vi "RT Variable Test.vi"() -> ()   [LabVIEW 2015]
panel:
  out "Log?":bool
  out "Operating?":bool
  out "a":dbl
  in  "stop":bool
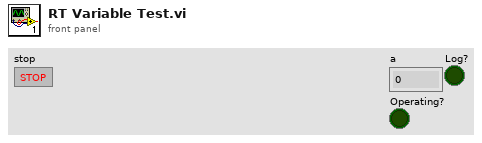
[diagram p1: front panel]
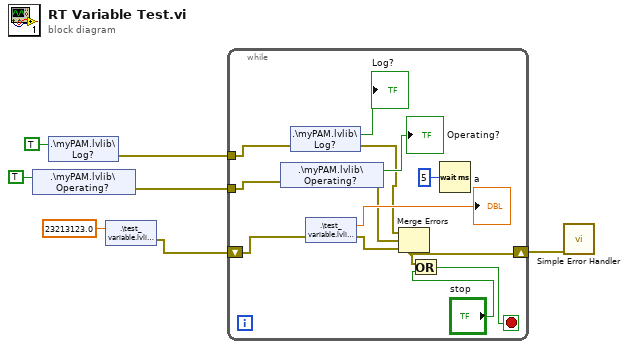
[diagram p0: block diagram]
diagram:
  n1 = shared-variable ".\\myPAM.lvlib\\Operating?"(TRUE ("Operating?")) -> (error out=w3:errorcluster)  [unwired: 1 in]
  n2 = shared-variable ".\\myPAM.lvlib\\Log?"(TRUE ("Log?")) -> (error out=w1:errorcluster)  [unwired: 1 in]
  n3 = shared-variable ".\\test_variable.lvlib\\a"(23213123.0 ("a")) -> (error out=w6:errorcluster)  [unwired: 1 in]
  n4 = while {
    tunnel: w3 -> [w15]
    tunnel: w1 -> [w11]
    shift-right: [w12] -> w7
    shift-left: w6 -> [w16]
    stop <- w17 stop-if-true
    n5 = shared-variable ".\\myPAM.lvlib\\Operating?"(error in=w15) -> (→"Operating?":bool, error out=w10:errorcluster)
    n6 = shared-variable ".\\myPAM.lvlib\\Log?"(error in=w11) -> (→"Log?":bool, error out=w8:errorcluster)
    n7 = shared-variable ".\\test_variable.lvlib\\a"(error in=w16) -> (→"a":dbl, error out=w13:errorcluster)
    n8 = Merge Errors(w8, w10, w13) -> (w12:errorcluster)
    n9 = Or(x=w12, y="stop") -> (x .or. y?=w17:bool)
    n10 = Wait (ms)(milliseconds to wait=u32 5) -> ()  [unwired: 1 out]
  }
  n11 = call <vilib>:"Simple Error Handler.vi"("error in (no error)"=w7) -> ()  [unwired: 4 in, 5 out]
